vi "ScaleTo_dBm_20190910.vi"(11 "Power Spectrum In (Volts)":dbl[](array[numeric])) -> (3 "P (dBm)":dbl[](array[numeric]))   [LabVIEW 2018]
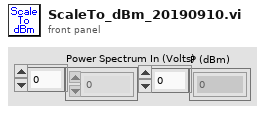
[diagram p1: front panel]
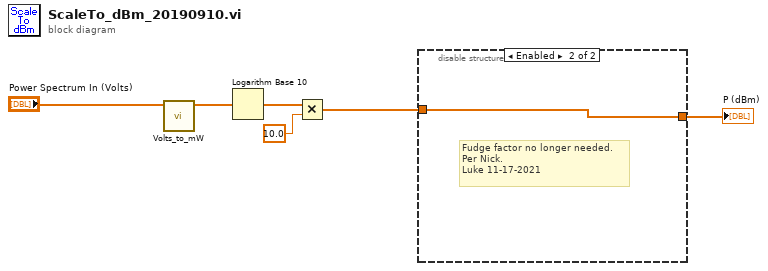
[diagram p0: block diagram]
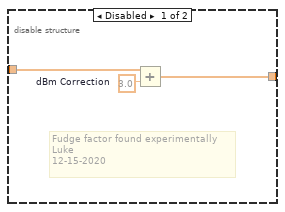
[diagram p2: hidden frame]
diagram:
  n1 = call "Volts_to_mW.vi"("Volts"="Power Spectrum In (Volts)") -> ("Power mW"=w1:dbl[])  [unwired: 10 in]
  n2 = Logarithm Base 10(1:w1) -> (0:w5:dbl[])
  n3 = Multiply(x=w5, y=10.0) -> (x*y=w4:dbl[])
  n4 = disable-structure shown="Enabled" {
    disable-tunnel: w4 -> [w8 w10]
    disable-tunnel: [w7 w10] -> w3
    frame Disabled {
      w9 = 3.0  # dBm Correction
      # "Fudge factor found experimentally\nLuke\n12-15-2020"
      n5 = Add(x=w8, y=w9) -> (x+y=w7:dbl[])
    }
    frame Enabled {
      # "Fudge factor no longer needed.\nPer Nick.\nLuke 11-17-2021"
    }
  }
  "P (dBm)" <- w3
